vi "Read Encoder Type.vi"(0 "class data in":refnum<class "MB_ENGINE.lvclass">, 11 "error in (no error)":errorcluster) -> (4 "class data out":refnum<class "MB_ENGINE.lvclass">, 6 "type":u16, 15 "error out":errorcluster)   [LabVIEW 2019, in "MB_ENGINE.lvclass"]
uses:
  MB_ENGINE.lvclass
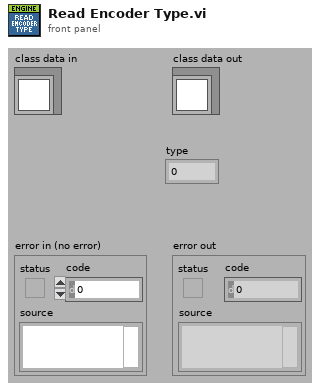
[diagram p1: front panel]
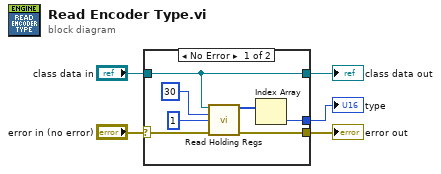
[diagram p0: block diagram]
diagram:
  n1 = case shown="No Error" "error in (no error)" {
    selector: "error in (no error)" -> [w9 w14]
    tunnel: [w8 w14] -> w4
    tunnel: "class data in" -> [w11 w13]
    tunnel: [w11 w13] -> w2
    tunnel: [w12 _] -> w1
    frame No Error {
      n2 = call-dynamic "Read Holding Regs.vi"("reference in"=w11, "starting address"=u16 30, "number of inputs"=u16 1, "error in (no error)"=w9) -> ("register values"=w10:u16[], "error out"=w8:errorcluster)  [unwired: 10 in]
      n3 = Index Array(array=w10) -> (element=w12:u16)  [unwired: 1 in]
    }
    frame Error {
    }
  }
  "error out" <- w4
  "class data out" <- w2
  "type" <- w1
